vi "Hochdruckregler_PID.vi"(0 "Regler Hochdruck":bool, 1 "PID Hochdruck":T1={"proportional gain (Kc)"=7.5000000000000036, "integral time (Ti, min)"=0.3499999999999999, "derivative time (Td, min)"=0.0} {"derivative time (Td, min)" format="%.3f"; "integral time (Ti, min)" format="%.3f"; "proportional gain (Kc)" format="%.3f"}, 2 "Dynamic Data":dynamicdata(waveform), 3 "upper limit in":dbl=70.0, 5 "lower limit":dbl=10.0, 7 "Hochdrucksteuerung":bool, 9 "Solldruck":dbl format="%.2f", 12 "PI05":dbl[](array[numeric]), 13 "Exp.V":dbl, 14 "reinitialize? (F) in":bool) -> (4 "Expansionsstellung":dbl, 6 "änderung expansion":dbl format="%.2f", 8 "upper limit out":dbl)   [LabVIEW 2015]
uses:
  <vilib>/addons/control/pid/pid.llb/PID (DBL).vi
  <vilib>/addons/control/pid/NI_PID_pid.lvlib
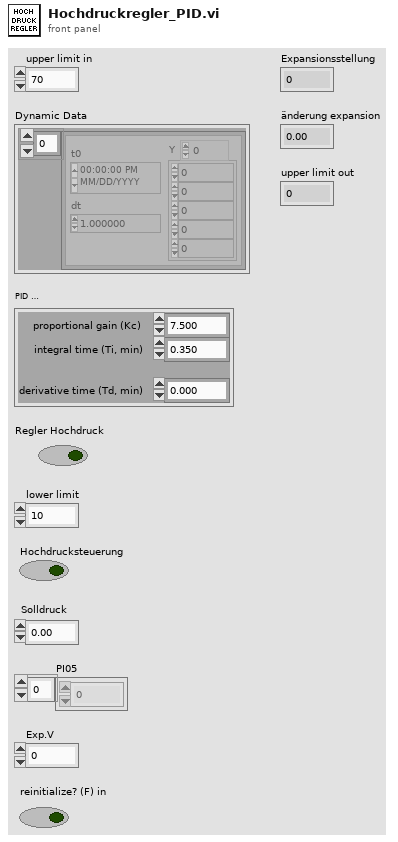
[diagram p1: front panel]
types:
  T1 = cluster{"proportional gain (Kc)":dbl, "integral time (Ti, min)":dbl, "derivative time (Td, min)":dbl}
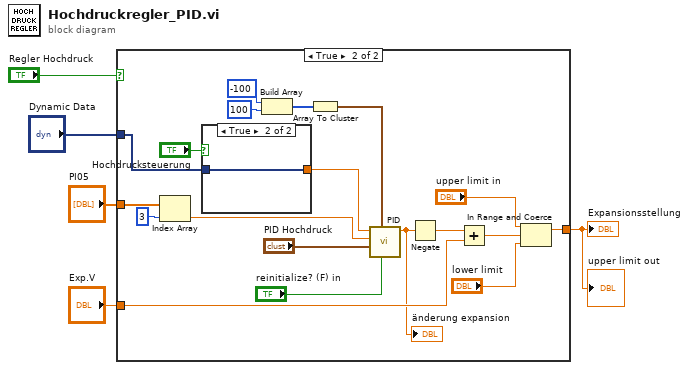
[diagram p0: block diagram]
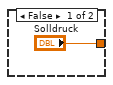
[diagram p3: hidden frame]
diagram:
  n1 = case shown="True" "Regler Hochdruck" {
    tunnel: "PI05" -> [_ w24]
    tunnel: "Exp.V" -> [w6 w16]
    tunnel: [w6 w15] -> w3
    tunnel: "Dynamic Data" -> [_ w7]
    frame False {
    }
    frame True {
      n2 = Index Array(array=w24, index=3) -> (element=w18:dbl)
      n3 = case shown="True" "Hochdrucksteuerung" {
        tunnel: ["Solldruck" w27] -> w17
        tunnel: w7 -> [_ w27]
        frame False {
        }
        frame True {
        }
      }
      n4 = Build Array(-100, 100) -> (w22:i32[])
      n5 = Array To Cluster(array=w22) -> (cluster=w19:cluster{"[0]":i32, "[1]":i32})
      n6 = call-poly <vilib>:"PID.vi"("reinitialize? (F)"="reinitialize? (F) in", "output range"=w19, "PID gains"="PID Hochdruck", "process variable"=w18, "setpoint"=w17) -> ("output"=w9:dbl)  [unwired: 5 in, 1 out]
      "änderung expansion" <- w9
      n7 = Negate(x=w9) -> (-x=w10:dbl)
      n8 = Add(x=w10, y=w16) -> (x+y=w14:dbl)
      n9 = In Range and Coerce(upper limit="upper limit in", x=w14, lower limit="lower limit") -> (coerced(x)=w15:dbl)  [unwired: 1 out]
    }
  }
  "Expansionsstellung" <- w3
  "upper limit out" <- w3
